vi "아날로그 out_연속샘플.vi"() -> ()   [LabVIEW 2018]
uses:
  <vilib>/DAQmx/write.llb/DAQmx Write (Analog Wfm 1Chan NSamp).vi
  <vilib>/DAQmx/create/channels.llb/DAQmx Create Channel (AO-Voltage-Basic).vi
  <vilib>/DAQmx/configure/timing.llb/DAQmx Timing (Sample Clock).vi
  <vilib>/DAQmx/miscellaneous.llb/DAQmx Fill In Error Info.vi
  <vilib>/measure/NI_MABase.lvlib
panel:
  in  "physical channels":tag caption="물리적 채널"
  in  "정지 버튼":bool
  out "signal out":waveform(dbl)(graph) caption="신호 출력"
  in  "signal type":T1(ring) caption="신호 타입"
  in  "amplitude":dbl=1.0 caption="amplitude [V]" format="%0.2p"
  in  "frequency":dbl=10.0 caption="주파수" format="%0.2p"
  out "error out":errorcluster caption="에러 출력"
  in  "samples per channel":i32=1000 caption="채널당 샘플"
  in  "sample mode":i32(ring)=10178 caption="샘플 모드" items=["유한 샘플"=10178, "연속 샘플"=10123, "하드웨어 타이밍에 의한 단일 포인트"=12522]
  in  "rate":dbl=1000.0 caption="속도" format="%0.2f"
  in  "channel name":string caption="할당된 이름"
  in  "minimum value":dbl=-5.0 caption="최소값" format="%0.2f"
  in  "maximum value":dbl=5.0 caption="최대값" format="%0.2f"
  in  "error in":errorcluster caption="에러 입력"
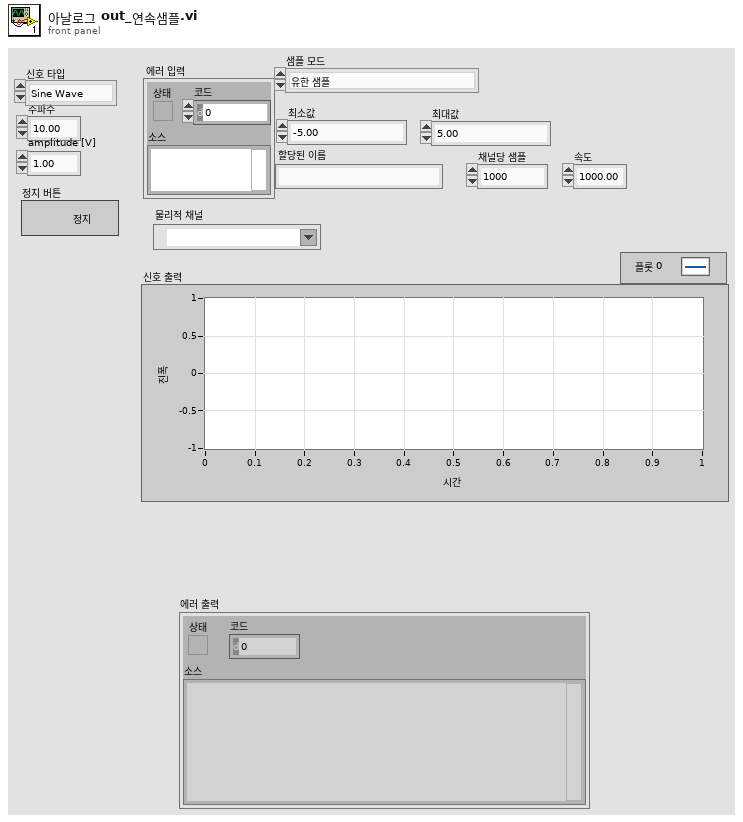
[diagram p1: front panel]
types:
  T1 = enum16{"Sine Wave", "Triangle Wave", "Square Wave", "Sawtooth Wave"}
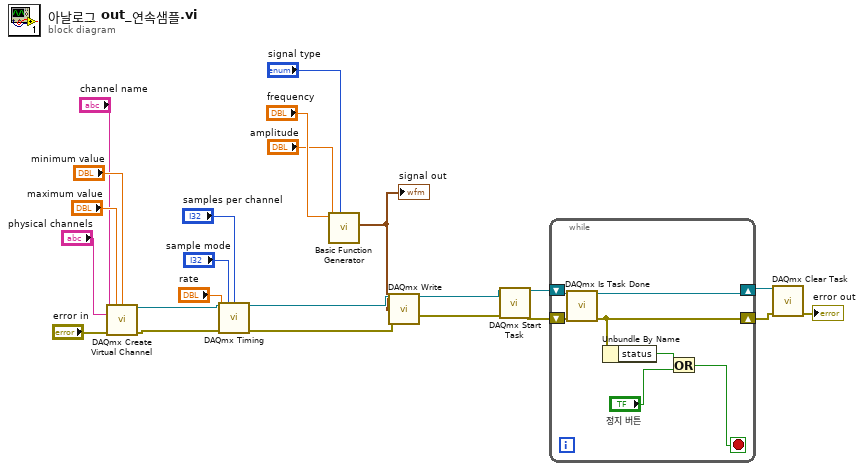
[diagram p0: block diagram]
diagram:
  n1 = call-poly <vilib>:"DAQmx Create Virtual Channel.vi"("maximum value"="maximum value", "minimum value"="minimum value", "physical channels"="physical channels", "name to assign"="channel name", "error in"="error in") -> ("task out"=w22:refnum<k21>, "error out"=w21:errorcluster)  [unwired: 9 in]
  n2 = call-poly <vilib>:"DAQmx Timing.vi"("task/channels in"=w22, "sample mode"="sample mode", "samples per channel"="samples per channel", "rate"="rate", "error in"=w21) -> ("task out"=w13:refnum<k21>, "error out"=w12:errorcluster)  [unwired: 9 in]
  n3 = call <vilib>:"Basic Function Generator.vi"("signal type"="signal type", "amplitude"="amplitude", "frequency"="frequency") -> ("signal out"=w8:waveform(dbl))  [unwired: 6 in, 2 out]
  "signal out" <- w8
  n4 = call-poly <vilib>:"DAQmx Write.vi"("task/channels in"=w13, "data"=w8, "error in"=w12) -> ("task out"=w7:refnum<k21>, "error out"=w6:errorcluster)  [unwired: 10 in, 1 out]
  n5 = call <vilib>:"DAQmx Start Task.vi"("task/channels in"=w7, "error in"=w6) -> ("task out"=w5:refnum<k21>, "error out"=w4:errorcluster)  [unwired: 12 in]
  n6 = while {
    shift-right: [w28] -> w3
    shift-left: w5 -> [w30]
    shift-right: [w27] -> w2
    shift-left: w4 -> [w29]
    stop <- w24 stop-if-true
    n7 = call <vilib>:"DAQmx Is Task Done.vi"("task/channels in"=w30, "error in"=w29) -> ("task out"=w28:refnum<k21>, "error out"=w27:errorcluster)  [unwired: 11 in, 1 out]
    n8 = Unbundle By Name(w27) -> ("status"=w25:bool)
    n9 = Or(x=w25, y="정지 버튼") -> (x .or. y?=w24:bool)
  }
  n10 = call <vilib>:"DAQmx Clear Task.vi"("task in"=w3, "error in"=w2) -> ("error out"=→"error out":errorcluster)  [unwired: 13 in]
